vi "2-2AAV.vi"() -> ()   [LabVIEW 2024]
panel:
  out "Waveform Graph 2":dynamicdata(graph)
  out "Average Value":dbl
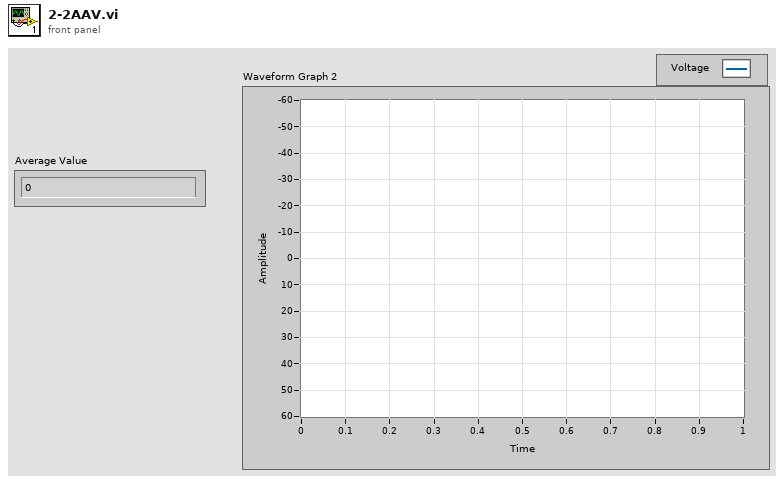
[diagram p1: front panel]
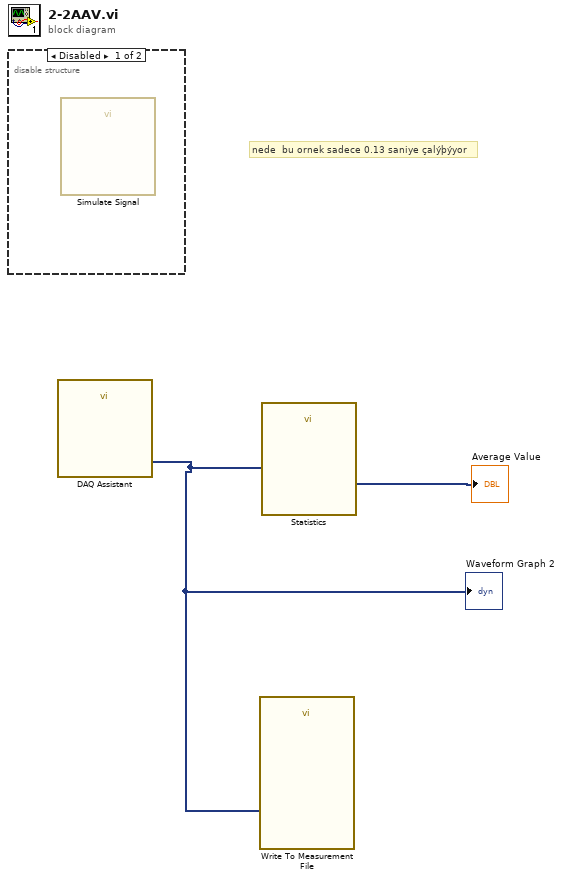
[diagram p0: block diagram]
diagram:
  # "nede  bu ornek sadece 0.13 saniye çalýþýyor"
  n1 = disable-structure shown="Disabled" {
    frame Disabled {
      n2 = call "Simulate Signal"() -> ()  [unwired: 14 in, 2 out]
    }
    frame Enabled {
    }
  }
  n3 = call "DAQ Assistant"() -> ("data"=w1:dynamicdata)  [unwired: 17 in, 2 out]
  "Waveform Graph 2" <- w1
  n4 = call "Write To Measurement File"("Signals"=w1) -> ()  [unwired: 16 in, 3 out]
  n5 = call "Statistics"("Signals"=w1) -> ("Arithmetic Mean"=→"Average Value":dynamicdata)  [unwired: 24 in, 2 out]
